vi "ProyectoIII.vi"() -> ()   [LabVIEW 2018]
panel:
  out "Numeric":i64
  out "MEMORY MAP":string[](array[string])
  out "Finished Job Table":string[][](table)
  out "USING DISK":string
  out "NEW":string[](array[string])
  out "RUNNING":string
  out "Program Control Block":string[][](table)
  in  "Address Probability (%)":i32(slide)=64 scale=0.0..100.0
  in  "Page Frames (KB)":i32(slide) step=4 scale=4.0..64.0
  in  "RAM (KB)":i32(slide)=64 step=4 scale=32.0..256.0
  out "WAITING DISK":string[](array[string])
  out "Table Allocation Page":string[][](table)
  in  "Play/Pause":bool
  in  "JOBS":i32=20
  out "I/O WAITING":string[](array[string])
  out "PRINT":string
  out "TERMINATED":string[](array[string])
  out "READY":string[](array[string])
  in  "?":bool
  in  "Delay (s)":sgl(slide) scale=0.0..6.0
  in  "Average Printing Time":i32(slide) scale=10.0..80.0
  in  "Print Probability %":i32(slide) scale=0.0..100.0
  in  "Average Process Time":i32(slide) scale=5.0..100.0
  in  "Quantum":i32(slide) scale=0.0..20.0
  in  "Job Probability %":i32(slide) scale=0.0..100.0
  out "Tiempo imprimiendo":i32
  out "quantum":i32
  out "CLOCK":i32
  # "MEMORY AND PROCESS MANAGER"
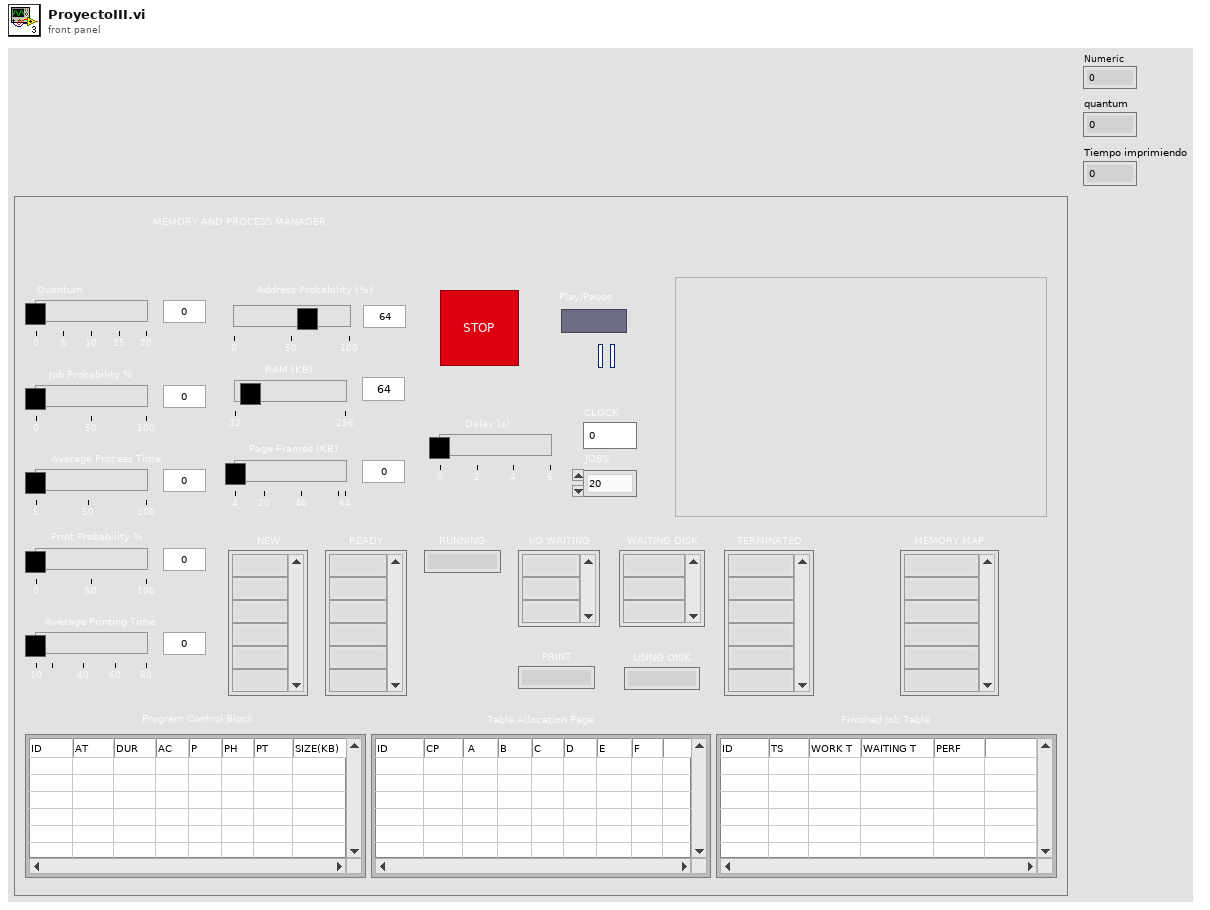
[diagram p1: front panel]
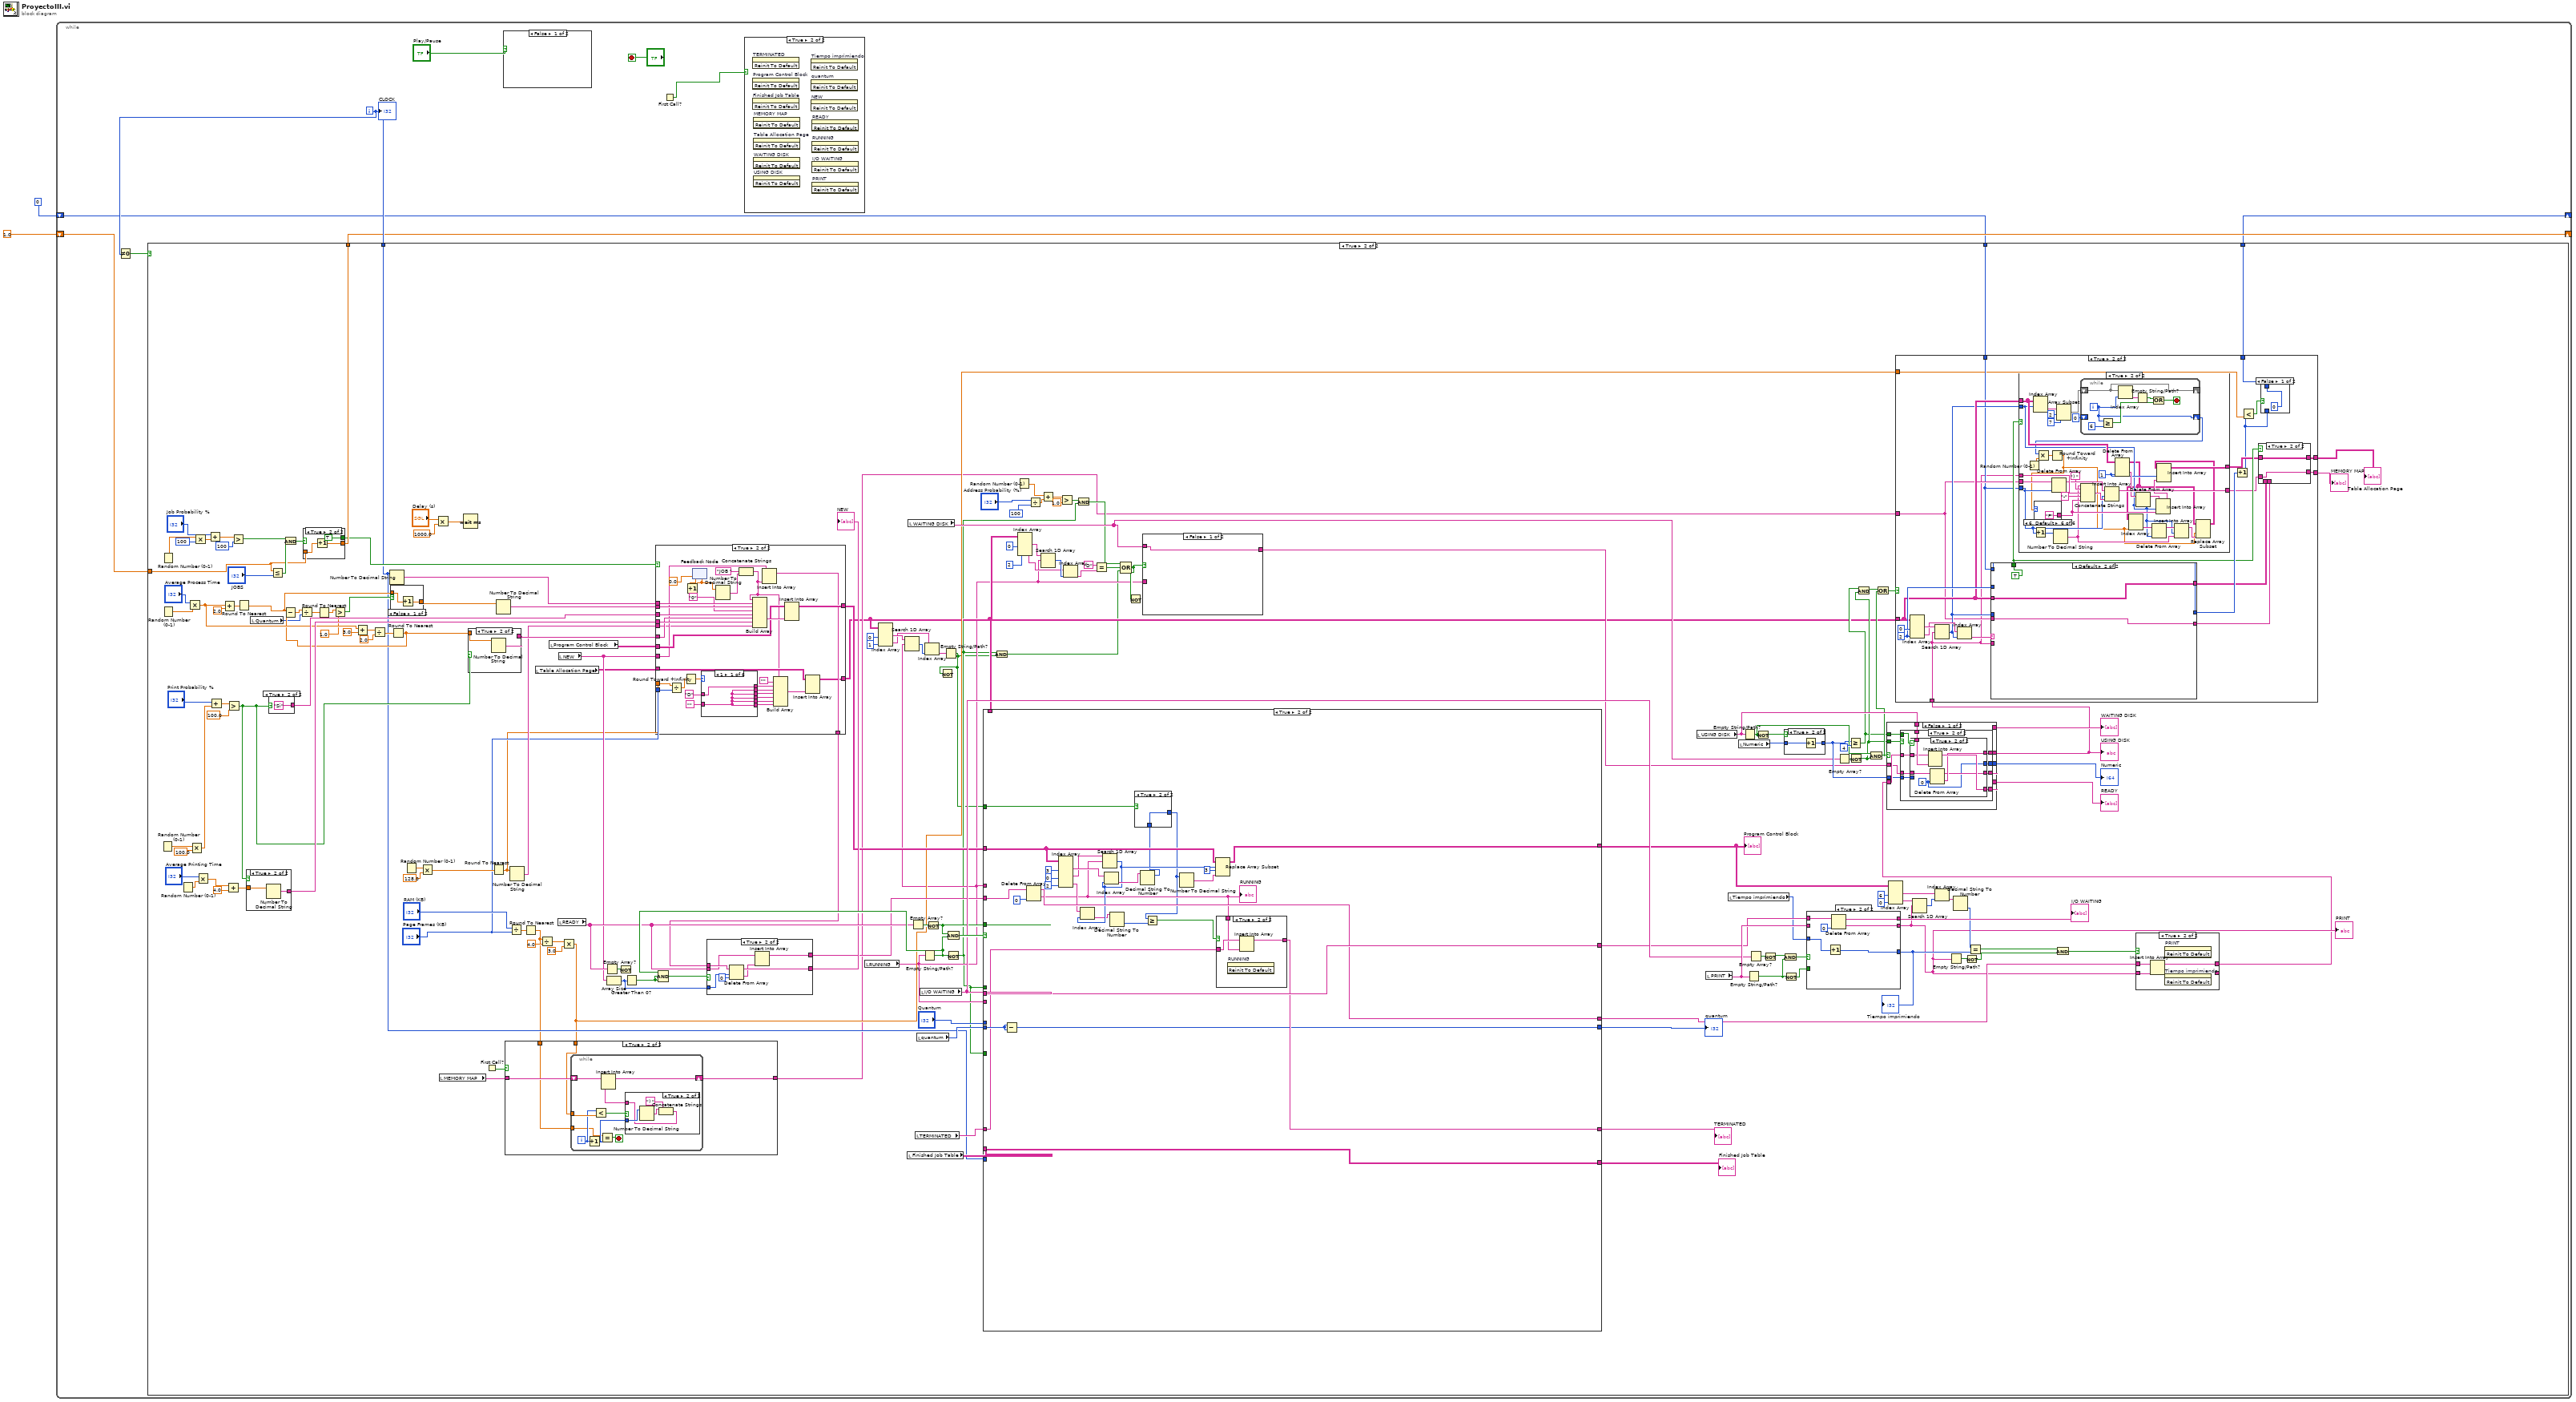
[diagram p0: block diagram]
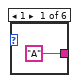
[diagram p8: hidden frame]
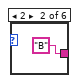
[diagram p9: hidden frame]
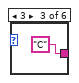
[diagram p10: hidden frame]
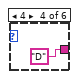
[diagram p11: hidden frame]
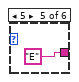
[diagram p12: hidden frame]
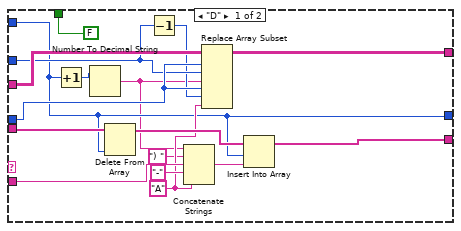
[diagram p13: hidden frame]
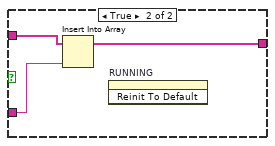
[diagram p14: hidden frame]
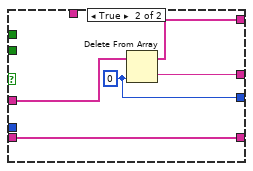
[diagram p17: hidden frame]
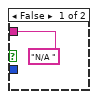
[diagram p20: hidden frame]
diagram:
  n1 = while {
    shift-right: [w6] -> _
    shift-left: 1.0 -> [w7]
    shift-right: [w4] -> _
    shift-left: 0 -> [w5]
    i -> [w8]
    stop <- "?" stop-if-true
    n2 = Not Equal To 0?(x=w8) -> (x != 0?=w9:bool)
    n3 = case shown="True" w9 {
      tunnel: w8 -> [_ w56]
      tunnel: w7 -> [_ w87]
      tunnel: [_ w86] -> w6
      tunnel: w5 -> [w12 w42]
      tunnel: [w12 w40] -> w4
      frame False {
      }
      frame True {
        n4 = Random Number (0-1)() -> (number: 0 to 1=w165:dbl)
        n5 = Random Number (0-1)() -> (number: 0 to 1=w168:dbl)
        n6 = Random Number (0-1)() -> (number: 0 to 1=w171:dbl)
        n7 = Random Number (0-1)() -> (number: 0 to 1=w170:dbl)
        n8 = Multiply(x="Average Process Time", y=w171) -> (x*y=w123:dbl)
        n9 = Multiply(x=w165, y=100.0) -> (x*y=w163:dbl)
        n10 = Multiply(x=w168, y=100) -> (x*y=w166:dbl)
        n11 = Multiply(x="Average Printing Time", y=w170) -> (x*y=w115:dbl)
        n12 = Add(x="Job Probability %", y=w166) -> (x+y=w92:dbl)
        n13 = Add(x="Print Probability %", y=w163) -> (x+y=w178:dbl)
        n14 = Add(x=w123, y=2.0) -> (x+y=w125:dbl)
        n15 = Add(x=w115, y=4.0) -> (x+y=w114:dbl)
        n16 = Greater?(x=w178, y=100.0) -> (0:w157:bool)
        n17 = Greater?(x=w92, y=100) -> (0:w89:bool)
        n18 = Round To Nearest(number=w125) -> (nearest integer value=w95:dbl)
        n19 = case shown="True" w157 {
          tunnel: w114 -> [_ w385]
          tunnel: ["" w384] -> w169
          frame False {
          }
          frame True {
            n20 = Number To Decimal String(number=w385) -> (decimal integer string=w384:string)  [unwired: 1 in]
          }
        }
        n21 = local read "Quantum"() -> (w101:i32)
        n22 = case shown="True" w157 {
          tunnel: ["No" "Si"] -> w172
          frame False {
          }
          frame True {
          }
        }
        n23 = Less Or Equal?(x=w87, y="JOBS") -> (x <= y?=w90:bool)
        n24 = And(x=w89, y=w90) -> (x .and. y?=w88:bool)
        n25 = case shown="True" w88 {
          tunnel: w87 -> [w345 w348]
          tunnel: [w345 w347] -> w86
          tunnel: [FALSE TRUE] -> w78
          frame False {
          }
          frame True {
            n26 = Increment(x=w348) -> (x+1=w347:dbl)
          }
        }
        n27 = Add(x=w123, y=3.0 ("x+y")) -> (x+y=w160:dbl)
        n28 = Divide(x=w160, y=2.0) -> (x/y=w158:dbl)
        n29 = Number To Decimal String(number=w56) -> (decimal integer string=w174:string)  [unwired: 1 in]
        n30 = Round To Nearest(number=w158) -> (nearest integer value=w102:dbl)
        n31 = Subtract(x=w95, y=w102) -> (x-y=w100:dbl)
        n32 = Divide(x=w100, y=w101) -> (x/y=w99:dbl)
        n33 = Round To Nearest(number=w99) -> (nearest integer value=w98:dbl)
        n34 = Greater?(x=w98, y=1.0) -> (0:w96:bool)
        n35 = case shown="False" w96 {
          tunnel: w95 -> [w349 w351]
          tunnel: [w350 w351] -> w94
          frame False {
            n36 = Increment(x=w349) -> (x+1=w350:dbl)
          }
          frame True {
          }
        }
        n37 = Random Number (0-1)() -> (number: 0 to 1=w85:dbl)
        n38 = Multiply(x=w85, y=128.0) -> (x*y=w83:dbl)
        n39 = Multiply(x="Delay (s)", y=1000.0 ("x*y")) -> (x*y=w175:dbl)
        n40 = local read "MEMORY MAP"() -> (w39:string[])
        n41 = Wait (ms)(milliseconds to wait=w175) -> ()  [unwired: 1 out]
        n42 = case shown="True" w157 {
          tunnel: ["" w382] -> w161
          tunnel: w102 -> [_ w381]
          frame False {
          }
          frame True {
            n43 = Number To Decimal String(number=w381) -> (decimal integer string=w382:string)  [unwired: 1 in]
          }
        }
        n44 = First Call?() -> (First Call?: T/F=w38:bool)
        n45 = Round To Nearest(number=w83) -> (nearest integer value=w76:dbl)
        n46 = Number To Decimal String(number=w94) -> (decimal integer string=w173:string)  [unwired: 1 in]
        n47 = Divide(x="RAM (KB)", y="Page Frames (KB)") -> (x/y=w79:dbl)
        n48 = Number To Decimal String(number=w76) -> (decimal integer string=w82:string)  [unwired: 1 in]
        n49 = Round To Nearest(number=w79) -> (nearest integer value=w29:dbl)
        n50 = local read "Table Allocation Page"() -> (w75:string[][])
        n51 = Divide(x=w29, y=4.0) -> (x/y=w32:dbl)
        n52 = local read "Program Control Block"() -> (w155:string[][])
        n53 = local read "READY"() -> (w107:string[])
        n54 = local read "NEW"() -> (w104:string[])
        n55 = Multiply(x=w32, y=3.0) -> (x*y=w27:dbl)
        n56 = case shown="True" w38 {
          tunnel: w39 -> [w325 w329]
          tunnel: [w325 w328] -> w25
          tunnel: w27 -> [_ w327]
          tunnel: w29 -> [_ w326]
          frame False {
          }
          frame True {
            n57 = while {
              tunnel: w327 -> [w336]
              shift-right: [w331] -> w328
              shift-left: w329 -> [w332]
              tunnel: w326 -> [w330]
              i -> [w334]
              stop <- w338 stop-if-true
              n58 = Increment(x=w334) -> (x+1=w333:i32)
              n59 = Less?(x=w334, y=w336) -> (x < y?=w335:bool)
              n60 = Equal?(x=w330, y=w333) -> (x = y?=w338:bool)
              n61 = case shown="True" w335 {
                tunnel: ["N/A " w340] -> w337
                tunnel: w333 -> [_ w343]
                frame False {
                }
                frame True {
                  n62 = Number To Decimal String(number=w343) -> (decimal integer string=w342:string)  [unwired: 1 in]
                  n63 = Concatenate Strings(w342, ") " ("string")) -> (w340:string)
                }
              }
              n64 = Insert Into Array(array=w332, new element=w337) -> (w331:string[])  [unwired: 1 in]
            }
          }
        }
        n65 = Empty Array?(array=w107) -> (empty?=w109:bool)
        n66 = Array Size(array=w104) -> (size(s)=w106:i32)
        n67 = Not(x=w109) -> ()  [unwired: 1 out]
        n68 = Greater Than 0?(x=w106) -> (x > 0?=w103:bool)
        n69 = case shown="True" w78 {
          tunnel: w174 -> [_ w417]
          tunnel: w173 -> [_ w416]
          tunnel: [w387 w421] -> w72
          tunnel: w172 -> [_ w414]
          tunnel: w169 -> [_ w413]
          tunnel: w161 -> [_ w412]
          tunnel: w155 -> [w387 w411]
          tunnel: w104 -> [w388 w409]
          tunnel: [w388 w408] -> w93
          tunnel: w82 -> [_ w406]
          tunnel: "Page Frames (KB)" -> [_ w404]
          tunnel: w76 -> [_ w403]
          tunnel: w75 -> [w386 w393]
          tunnel: [w386 w391] -> w23
          frame False {
          }
          frame True {
            n70 = Divide(x=w403, y=w404) -> (x/y=w405:dbl)
            n71 = Round Toward +Infinity(x=w405) -> (ceil(x): smallest int >= x=w401:dbl)
            n72 = feedback #1(0.0) -> (w418:dbl)
            n73 = Increment(x=w418) -> (x+1=w419:dbl)
            n74 = feedback-in #1(w419) -> ()
            n75 = case shown="1" w401 {
              tunnel: [w424 w426 w428 w430 w432 w433] -> w390
              tunnel: "D" -> [w424 w426 w428 w430 w432 w433]
              tunnel: "" -> [w423 w425 w427 w429 w431 _]
              tunnel: [w423 w425 w427 w429 w432 w433] -> w395
              tunnel: [w423 w426 w428 w430 w432 w433] -> w398
              tunnel: [w423 w425 w428 w430 w432 w433] -> w397
              tunnel: [w423 w425 w427 w430 w432 w433] -> w396
              tunnel: [w423 w425 w427 w429 w431 w433] -> w394
              frame 1 {
              }
              frame 2 {
              }
              frame 3 {
              }
              frame 4 {
              }
              frame 5 {
              }
              frame 6, Default {
              }
            }
            n76 = Number To Decimal String(number=w418) -> (decimal integer string=w410:string)  [unwired: 1 in]
            n77 = Concatenate Strings("JOB ", w410) -> (w392:string)
            n78 = Build Array(w392, w417, w416, "0", w414, w412, w413, w406) -> (w422:string[])
            n79 = Insert Into Array(array=w409, new element=w392) -> (w408:string[])  [unwired: 1 in]
            n80 = Build Array(w392, "", w390, w398, w397, w396, w395, w394) -> (w402:string[])
            n81 = Insert Into Array(array=w411, new element=w422) -> (w421:string[][])  [unwired: 2 in]
            n82 = Insert Into Array(array=w393, new element=w402) -> (w391:string[][])  [unwired: 2 in]
          }
        }
        n83 = local read "RUNNING"() -> (w19:string)
        n84 = Index Array(array=w23, index (col) #1=0 ("disabled index (col)"), index (col) #2=1 ("index (col)")) -> (element #1=w20:string[], element #2=w17:string[])  [unwired: 2 in]
        n85 = Search 1D Array(1D array=w20, element=w19) -> (index of element=w18:i32)  [unwired: 1 in]
        n86 = local read "Finished Job Table"() -> (w112:string[][])
        n87 = local read "WAITING DISK"() -> (w47:string[])
        n88 = Empty Array?(array=w107) -> (empty?=w162:bool)
        n89 = local read "TERMINATED"() -> (w127:string[])
        n90 = local read "quantum"() -> (w145:i32)
        n91 = local read "I/O WAITING"() -> (w150:string[])
        n92 = Empty String/Path?(string/path=w19) -> (empty?=w108:bool)
        n93 = Compound Arithmetic op=AND(w108, w103, w103) -> (w110:bool)
        n94 = case shown="True" w110 {
          tunnel: w107 -> [w352 w356]
          tunnel: w93 -> [w353 w360]
          tunnel: w106 -> [_ w359]
          tunnel: [w353 w358] -> w105
          tunnel: [w352 w355] -> w67
          frame False {
          }
          frame True {
            n95 = Delete From Array(array=w360, length=w359, index=0) -> (deleted portion=w357:string[], array with subset deleted=w358:string[])
            n96 = Insert Into Array(array=w356, new element=w357) -> (w355:string[])  [unwired: 1 in]
          }
        }
        "NEW" <- w105
        n97 = Index Array(array=w17, index=w18) -> (element=w16:string)
        n98 = Not(x=w162) -> (.not. x?=w147:bool)
        n99 = Empty String/Path?(string/path=w16) -> (empty?=w13:bool)
        n100 = Not(x=w13) -> ()  [unwired: 1 out]
        n101 = Not(x=w108) -> (.not. x?=w15:bool)
        n102 = Compound Arithmetic op=AND(w147, w108) -> (w156:bool)
        n103 = case shown="True" w156 {
          tunnel: w67 -> [w479 w602]
          tunnel: w19 -> [w485 _]
          tunnel: w72 -> [w463 w594]
          tunnel: [w462 w593] -> w81
          tunnel: w150 -> [w486 w592]
          tunnel: [w484 w592] -> w149
          tunnel: w15 -> [w480 _]
          tunnel: [w438 w591] -> w128
          tunnel: w19 -> [w436 _]
          tunnel: w145 -> [w443 w590]
          tunnel: "Quantum" -> [w477 _]
          tunnel: [w474 w579] -> w146
          tunnel: w15 -> [w478 _]
          tunnel: w147 -> [w476 _]
          tunnel: w127 -> [w468 w583]
          tunnel: [w467 w582] -> w126
          tunnel: w112 -> [w460 w581]
          tunnel: w56 -> [w459 _]
          tunnel: [w456 w581] -> w111
          tunnel: w23 -> [_ _]
          tunnel: w13 -> [_ w578]
          frame False {
            n104 = Increment(x=w443) -> (x+1=w444:i32)
            n105 = Less Or Equal?(x=w477, y=w444) -> (x <= y?=w461:bool)
            n106 = Index Array(array=w463, index (col) #1=0 ("disabled index (col)"), index (col) #2=3 ("index (col)")) -> (element #1=w501:string[], element #2=w500:string[])  [unwired: 2 in]
            n107 = Search 1D Array(1D array=w501, element=w485) -> (index of element=w497:i32)  [unwired: 1 in]
            n108 = Index Array(array=w500, index=w497) -> (element=w499:string)
            n109 = Decimal String To Number(string=w499) -> (number=w442:i32)  [unwired: 2 in, 1 out]
            n110 = Empty String/Path?(string/path=w436) -> (empty?=w466:bool)
            n111 = Increment(x=w442) -> (x+1=w440:i32)
            n112 = Not(x=w466) -> (.not. x?=w465:bool)
            n113 = Number To Decimal String(number=w440) -> (decimal integer string=w496:string)  [unwired: 1 in]
            n114 = Replace Array Subset(array=w463, new element=w496, index (row)=w497, index (col)=3 ("disabled index (col)")) -> (w462:string[][])
            n115 = Index Array(array=w462, index (col) #1=3 ("disabled index (col)"), index (col) #2=0 ("index (col)"), index (col) #3=2 ("index (col)"), index (col) #4=6 ("index (col)"), index (col) #5=1 ("index (col)")) -> (element #1=w470:string[], element #2=w471:string[], element #3=w454:string[], element #4=w453:string[], element #5=w451:string[])  [unwired: 5 in]
            n116 = Index Array(array=w462, index (col) #1=3 ("disabled index (col)"), index (col) #2=0 ("disabled index (col)"), index (col) #3=5 ("index (col)")) -> (element #1=w493:string[], element #2=w482:string[], element #3=w483:string[])  [unwired: 3 in]
            n117 = Search 1D Array(1D array=w482, element=w485) -> (index of element=w489:i32)  [unwired: 1 in]
            n118 = Search 1D Array(1D array=w471, element=w436) -> (index of element=w445:i32)  [unwired: 1 in]
            n119 = Index Array(array=w454, index=w445) -> (element=w441:string)
            n120 = Index Array(array=w470, index=w445) -> (element=w439:string)
            n121 = Index Array(array=w483, index=w489) -> (element=w488:string)
            n122 = Index Array(array=w493, index=w489) -> (element=w492:string)
            n123 = Decimal String To Number(string=w488) -> (number=w487:i32)  [unwired: 2 in, 1 out]
            n124 = Decimal String To Number(string=w492) -> (number=w491:i32)  [unwired: 2 in, 1 out]
            n125 = Equal?(x=w439, y=w441) -> (x = y?=w464:bool)
            n126 = Equal?(x=w487, y=w491) -> (x = y?=w475:bool)
            n127 = Compound Arithmetic op=AND(w464, w465) -> (w437:bool)
            n128 = Not(x=w437) -> (.not. x?=w448:bool)
            n129 = Compound Arithmetic op=AND(w461, w448) -> (w447:bool)
            n130 = Not(x=w447) -> (.not. x?=w446:bool)
            n131 = case shown="True" w447 {
              tunnel: w436 -> [_ w571]
              tunnel: w479 -> [w560 w570]
              tunnel: [w560 w569] -> w438
              tunnel: w476 -> [w562 _]
              tunnel: w478 -> [w559 _]
              tunnel: w443 -> [w558 w568]
              tunnel: [w557 w567] -> w474
              frame False {
                n132 = And(x=w562, y=w559) -> (x .and. y?=w561:bool)
                n133 = case shown="False" w561 {
                  tunnel: w558 -> [w564 w566]
                  tunnel: [w563 w565] -> w557
                  frame False {
                    n134 = Subtract(x=w564, y=w564) -> (x-y=w563:i32)
                  }
                  frame True {
                    n135 = Increment(x=w566) -> (x+1=w565:i32)
                  }
                }
              }
              frame True {
                n136 = Insert Into Array(array=w570, new element=w571) -> (w569:string[])  [unwired: 1 in]
                n137 = Subtract(x=w568, y=w568) -> (x-y=w567:i32)
              }
            }
            n138 = Compound Arithmetic op=AND(w475, w480, w448, w446) -> (w449:bool)
            n139 = case shown="True" w437 {
              tunnel: w468 -> [w534 w556]
              tunnel: w436 -> [w531 w535]
              tunnel: [w534 w555] -> w467
              tunnel: w460 -> [w533 w539]
              tunnel: w459 -> [_ w554]
              tunnel: w451 -> [_ w553]
              tunnel: w445 -> [_ w552]
              tunnel: w441 -> [w532 w537]
              tunnel: w453 -> [_ w546]
              tunnel: w445 -> [_ w545]
              tunnel: [w533 w540] -> w457
              tunnel: [w532 w537] -> w455
              tunnel: [w531 w535] -> w450
              tunnel: w436 -> [_ _]
              frame False {
              }
              frame True {
                w536 = "" ("element")
                n140 = Index Array(array=w546, index=w545) -> (element=w544:string)
                n141 = Decimal String To Number(string=w537) -> (number=w547:i32)  [unwired: 2 in, 1 out]
                n142 = Index Array(array=w553, index=w552) -> (element=w551:string)
                n143 = Insert Into Array(array=w556, new element=w535) -> (w555:string[])  [unwired: 1 in]
                n144 = Decimal String To Number(string=w544) -> (number=w543:i32)  [unwired: 2 in, 1 out]
                n145 = Decimal String To Number(string=w551) -> (number=w550:i32)  [unwired: 2 in, 1 out]
                n146 = Add(x=w547, y=w543) -> (x+y=w542:i32)
                n147 = Subtract(x=w554, y=w550) -> (x-y=w549:i32)
                n148 = Number To Decimal String(number=w542) -> (decimal integer string=w541:string)  [unwired: 1 in]
                n149 = Number To Decimal String(number=w549) -> (decimal integer string=w548:string)  [unwired: 1 in]
                n150 = Build Array(w535, w548, w541, w536, w536) -> (w538:string[])
                n151 = Insert Into Array(array=w539, new element=w538) -> (w540:string[][])  [unwired: 2 in]
              }
            }
            n152 = case shown="True" w449 {
              tunnel: w486 -> [w572 w575]
              tunnel: w485 -> [_ w574]
              tunnel: [w572 w573] -> w484
              frame False {
              }
              frame True {
                n153 = Insert Into Array(array=w575, new element=w574) -> (w573:string[])  [unwired: 1 in]
              }
            }
            n154 = Compound Arithmetic op=OR(w475, w447, w437) -> (w481:bool)
            n155 = case shown="True" w481 {
              frame False {
              }
              frame True {
                n156 = invoke on="RUNNING" class="Str" method="Reinit To Default"() -> ()  [unwired: 3 in, 3 out]
              }
            }
            n157 = case shown="True" w437 {
              tunnel: w457 -> [w504 w529]
              tunnel: [w504 w518] -> w456
              tunnel: w455 -> [_ w530]
              tunnel: w450 -> [_ w527]
              frame False {
              }
              frame True {
                n158 = Decimal String To Number(string=w530) -> (number=w522:i32)  [unwired: 2 in, 1 out]
                n159 = Index Array(array=w529, index (col) #1=1 ("disabled index (col)"), index (col) #2=0 ("index (col)"), index (col) #3=2 ("index (col)")) -> (element #1=w524:string[], element #2=w525:string[], element #3=w516:string[])  [unwired: 3 in]
                n160 = Search 1D Array(1D array=w525, element=w527) -> (index of element=w511:i32)  [unwired: 1 in]
                n161 = Index Array(array=w516, index=w511) -> (element=w515:string)
                n162 = Index Array(array=w524, index=w511) -> (element=w523:string)
                n163 = Decimal String To Number(string=w515) -> (number=w514:i32)  [unwired: 2 in, 1 out]
                n164 = Decimal String To Number(string=w523) -> (number=w513:i32)  [unwired: 2 in, 1 out]
                n165 = Divide(x=w514, y=w513) -> (x/y=w510:dbl)
                n166 = Subtract(x=w513, y=w522) -> (x-y=w521:i32)
                n167 = Multiply(x=w510, y=100.0) -> (x*y=w508:dbl)
                n168 = Number To Decimal String(number=w521) -> (decimal integer string=w520:string)  [unwired: 1 in]
                n169 = Number To Decimal String(number=w508) -> (decimal integer string=w507:string)  [unwired: 1 in]
                n170 = Concatenate Strings(w507, " %" ("string")) -> (w505:string)
                n171 = Replace Array Subset(array=w529, new element #1=w520, index (row) #1=w511, index (col) #1=3 ("disabled index (col)"), new element #2=w505, index (row) #2=w511, index (col) #2=4 ("index (col)")) -> (w518:string[][])
              }
            }
          }
          frame True {
            n172 = Subtract(x=w590, y=w590) -> (x-y=w579:i32)
            n173 = Delete From Array(array=w602, index=0) -> (deleted portion=w580:string, array with subset deleted=w591:string[])  [unwired: 1 in]
            "RUNNING" <- w580
            n174 = Index Array(array=w594, index (col) #1=3 ("disabled index (col)"), index (col) #2=0 ("index (col)"), index (col) #3=2 ("index (col)")) -> (element #1=w599:string[], element #2=w598:string[], element #3=w588:string[])  [unwired: 3 in]
            n175 = Search 1D Array(1D array=w598, element=w580) -> (index of element=w587:i32)  [unwired: 1 in]
            n176 = Index Array(array=w588, index=w587) -> (element=w586:string)
            n177 = Index Array(array=w599, index=w587) -> (element=w597:string)
            n178 = Decimal String To Number(string=w586) -> (number=w585:i32)  [unwired: 2 in, 1 out]
            n179 = Decimal String To Number(string=w597) -> (offset past number=w577:i32)  [unwired: 2 in, 1 out]
            n180 = case shown="True" w578 {
              tunnel: w577 -> [w604 w606]
              tunnel: [w605 w606] -> w576
              frame False {
                n181 = Increment(x=w604) -> (x+1=w605:i32)
              }
              frame True {
              }
            }
            n182 = Greater Or Equal?(x=w576, y=w585) -> (x >= y?=w584:bool)
            n183 = Number To Decimal String(number=w576) -> (decimal integer string=w595:string)  [unwired: 1 in]
            n184 = Replace Array Subset(array=w594, new element=w595, index (row)=w587, index (col)=3 ("disabled index (col)")) -> (w593:string[][])
            n185 = case shown="True" w584 {
              tunnel: w583 -> [w607 w610]
              tunnel: w580 -> [_ w609]
              tunnel: [w607 w608] -> w582
              frame False {
              }
              frame True {
                n186 = invoke on="RUNNING" class="Str" method="Reinit To Default"() -> ()  [unwired: 3 in, 3 out]
                n187 = Insert Into Array(array=w610, new element=w609) -> (w608:string[])  [unwired: 1 in]
              }
            }
          }
        }
        "Program Control Block" <- w81
        "quantum" <- w146
        "TERMINATED" <- w126
        "Finished Job Table" <- w111
        n188 = And(x=w15, y=w13) -> (x .and. y?=w14:bool)
        n189 = Random Number (0-1)() -> (number: 0 to 1=w74:dbl)
        n190 = Index Array(array=w23, index (col) #1=0 ("index (col)"), index (col) #2=2 ("index (col)")) -> (element #1=w51:string[], element #2=w52:string[])  [unwired: 2 in]
        n191 = Divide(x="Address Probability (%)", y=100) -> (x/y=w69:dbl)
        n192 = Add(x=w74, y=w69) -> (x+y=w73:dbl)
        n193 = Search 1D Array(1D array=w51, element=w19) -> (index of element=w53:i32)  [unwired: 1 in]
        n194 = Greater?(x=w73, y=1.0) -> (0:w46:bool)
        n195 = Index Array(array=w52, index=w53) -> (element=w54:string)
        n196 = And(x=w46, y=w15) -> (x .and. y?=w45:bool)
        n197 = Equal?(x="D", y=w54) -> (x = y?=w44:bool)
        n198 = Compound Arithmetic op=OR(w45, w44, w14) -> (w24:bool)
        n199 = Not(x=w24) -> ()  [unwired: 1 out]
        n200 = case shown="False" w24 {
          tunnel: w19 -> [_ w282]
          tunnel: [w279 w281] -> w48
          tunnel: w47 -> [w279 w280]
          frame False {
          }
          frame True {
            n201 = Insert Into Array(array=w280, new element=w282) -> (w281:string[])  [unwired: 1 in]
            n202 = invoke on="RUNNING" class="Str" method="Reinit To Default"() -> ()  [unwired: 3 in, 3 out]
          }
        }
        n203 = local read "USING DISK"() -> (w60:string)
        n204 = local read "PRINT"() -> (w151:string)
        n205 = local read "Tiempo imprimiendo"() -> (w144:i32)
        n206 = local read "Numeric"() -> (w65:i64)
        n207 = Empty String/Path?(string/path=w60) -> (empty?=w61:bool)
        n208 = Empty String/Path?(string/path=w151) -> (empty?=w134:bool)
        n209 = Empty Array?(array=w150) -> (empty?=w153:bool)
        n210 = Not(x=w61) -> (.not. x?=w34:bool)
        n211 = Not(x=w153) -> (.not. x?=w152:bool)
        n212 = And(x=w152, y=w134) -> (x .and. y?=w135:bool)
        n213 = case shown="True" w34 {
          tunnel: w65 -> [w322 w324]
          tunnel: [w322 w323] -> w57
          frame False {
          }
          frame True {
            n214 = Increment(x=w324) -> (x+1=w323:i64)
          }
        }
        n215 = Not(x=w134) -> (.not. x?=w133:bool)
        n216 = case shown="True" w135 {
          tunnel: w149 -> [w369 w379]
          tunnel: [w370 w378] -> w116
          tunnel: w151 -> [w370 _]
          tunnel: [w369 w377] -> w148
          tunnel: w144 -> [w367 w375]
          tunnel: [w366 w374] -> w136
          tunnel: w133 -> [w368 _]
          frame False {
            n217 = case shown="True" w368 {
              tunnel: w367 -> [w371 w373]
              tunnel: [w371 w372] -> w366
              frame False {
              }
              frame True {
                n218 = Increment(x=w373) -> (x+1=w372:i32)
              }
            }
          }
          frame True {
            n219 = Increment(x=w375) -> (x+1=w374:i32)
            n220 = Delete From Array(array=w379, index=0) -> (deleted portion=w378:string, array with subset deleted=w377:string[])  [unwired: 1 in]
          }
        }
        "I/O WAITING" <- w148
        "PRINT" <- w116
        "Tiempo imprimiendo" <- w136
        n221 = Empty Array?(array=w47) -> (empty?=w66:bool)
        n222 = Greater Or Equal?(x=w57, y=i64 4) -> (x >= y?=w26:bool)
        n223 = Not(x=w66) -> (.not. x?=w33:bool)
        n224 = Compound Arithmetic op=AND(w26, w33) -> (w37:bool)
        n225 = And(x=w61, y=w33) -> (x .and. y?=w36:bool)
        n226 = Or(x=w36, y=w37) -> (x .or. y?=w35:bool)
        n227 = Index Array(array=w81, index (col) #1=6 ("disabled index (col)"), index (col) #2=0 ("index (col)")) -> (element #1=w139:string[], element #2=w141:string[])  [unwired: 2 in]
        n228 = Search 1D Array(1D array=w141, element=w116) -> (index of element=w140:i32)  [unwired: 1 in]
        n229 = Index Array(array=w139, index=w140) -> (element=w138:string)
        n230 = Empty String/Path?(string/path=w116) -> (empty?=w132:bool)
        n231 = Decimal String To Number(string=w138) -> (number=w137:i32)  [unwired: 2 in, 1 out]
        n232 = Not(x=w132) -> (.not. x?=w129:bool)
        n233 = Equal?(x=w137, y=w136) -> (x = y?=w131:bool)
        n234 = And(x=w131, y=w129) -> (x .and. y?=w130:bool)
        n235 = case shown="True" w130 {
          tunnel: w128 -> [w362 w365]
          tunnel: w116 -> [w361 w364]
          tunnel: [w362 w363] -> w59
          tunnel: [w361 _] -> _
          frame False {
          }
          frame True {
            n236 = Insert Into Array(array=w365, new element=w364) -> (w363:string[])  [unwired: 1 in]
            n237 = invoke on="PRINT" class="Str" method="Reinit To Default"() -> ()  [unwired: 3 in, 3 out]
            n238 = invoke on="Tiempo imprimiendo" class="DigNum (strict)" method="Reinit To Default"() -> ()  [unwired: 3 in, 3 out]
          }
        }
        n239 = case shown="False" w36 {
          tunnel: w48 -> [w287 w321]
          tunnel: [w286 w320] -> w43
          tunnel: [w285 w319] -> w63
          tunnel: [w284 w318] -> w62
          tunnel: w33 -> [w292 _]
          tunnel: w26 -> [w291 _]
          tunnel: w60 -> [w290 _]
          tunnel: w59 -> [w289 w317]
          tunnel: [w288 w317] -> w58
          tunnel: w57 -> [w283 _]
          frame False {
            n240 = case shown="True" w292 {
              tunnel: w291 -> [_ w305]
              tunnel: w290 -> [w294 w304]
              tunnel: w289 -> [w295 w303]
              tunnel: [w295 w302] -> w288
              tunnel: w287 -> [w296 w301]
              tunnel: [w294 w300] -> w286
              tunnel: [w296 w299] -> w285
              tunnel: [w293 w298] -> w284
              tunnel: w283 -> [w293 w297]
              frame False {
              }
              frame True {
                n241 = case shown="True" w305 {
                  tunnel: w304 -> [w309 w316]
                  tunnel: w303 -> [w308 w315]
                  tunnel: [w308 w314] -> w302
                  tunnel: w301 -> [w307 w313]
                  tunnel: [w309 w312] -> w300
                  tunnel: [w307 w311] -> w299
                  tunnel: [w306 w310] -> w298
                  tunnel: w297 -> [w306 _]
                  frame False {
                  }
                  frame True {
                    w310 = 0 ("index")
                    n242 = Insert Into Array(array=w315, new element=w316) -> (w314:string[])  [unwired: 1 in]
                    n243 = Delete From Array(array=w313, index=w310) -> (deleted portion=w312:string, array with subset deleted=w311:string[])  [unwired: 1 in]
                  }
                }
              }
            }
          }
          frame True {
            w318 = 0 ("index")
            n244 = Delete From Array(array=w321, index=w318) -> (deleted portion=w320:string, array with subset deleted=w319:string[])  [unwired: 1 in]
          }
        }
        "READY" <- w58
        "USING DISK" <- w43
        "WAITING DISK" <- w63
        "Numeric" <- w62
        n245 = case shown="True" w35 {
          tunnel: w23 -> [w180 w198]
          tunnel: w43 -> [_ w189]
          tunnel: w42 -> [w181 w190]
          tunnel: w25 -> [w182 w191]
          tunnel: [w182 w187] -> w41
          tunnel: [w181 w184] -> w40
          tunnel: [w180 w194] -> w28
          tunnel: w27 -> [_ w183]
          frame False {
          }
          frame True {
            w200 = 2 ("index (col)")
            n246 = Index Array(array=w198, index (col) #1=0 ("disabled index (col)"), index (col) #2=w200) -> (element #1=w202:string[], element #2=w201:string[])  [unwired: 2 in]
            n247 = Search 1D Array(1D array=w202, element=w189) -> (index of element=w197:i32)  [unwired: 1 in]
            n248 = Index Array(array=w201, index=w197) -> (element=w203:string)
            n249 = case shown="Default" w203 {
              tunnel: w198 -> [w268 w278]
              tunnel: [w267 w278] -> w193
              tunnel: w190 -> [w260 w276]
              tunnel: w191 -> [w272 w277]
              tunnel: w189 -> [w274 _]
              tunnel: [w270 w277] -> w192
              tunnel: [w260 w276] -> w199
              tunnel: w197 -> [w266 _]
              tunnel: w200 -> [w265 _]
              tunnel: [FALSE TRUE] -> w196
              frame "D" {
                w261 = "A" ("string")
                n250 = Increment(x=w260) -> (x+1=w262:i32)
                n251 = Number To Decimal String(number=w262) -> (decimal integer string=w259:string)  [unwired: 1 in]
                n252 = Delete From Array(array=w272, index=w260) -> (array with subset deleted=w269:string[])  [unwired: 1 in, 1 out]
                n253 = Decrement(x=w265) -> (x-1=w264:i32)
                n254 = Concatenate Strings(w259, ") " ("string"), w274, "-" ("string"), w261) -> (w271:string)
                n255 = Replace Array Subset(array=w268, new element #1=w259, index (row) #1=w266, index (col) #1=w265, new element #2=w261, index (row) #2=w266, index (col) #2=w264) -> (w267:string[][])
                n256 = Insert Into Array(array=w269, index=w260, new element=w271) -> (w270:string[])
              }
              frame Default {
              }
            }
            n257 = case shown="True" w196 {
              tunnel: w198 -> [w212 w239]
              tunnel: w197 -> [_ w220]
              tunnel: [w212 w233] -> w195
              tunnel: w191 -> [w211 w236]
              tunnel: w190 -> [_ w216]
              tunnel: w189 -> [_ w237]
              tunnel: [w211 w234] -> w188
              frame False {
              }
              frame True {
                w231 = 1 ("disabled index (col)")
                n258 = Random Number (0-1)() -> (number: 0 to 1=w241:dbl)
                n259 = Index Array(array=w239, index (row)=w220) -> (element=w244:string[])  [unwired: 1 in]
                n260 = Increment(x=w216) -> (x+1=w229:i32)
                n261 = Delete From Array(array=w236, index=w216) -> (array with subset deleted=w230:string[])  [unwired: 1 in, 1 out]
                n262 = Number To Decimal String(number=w229) -> (decimal integer string=w215:string)  [unwired: 1 in]
                n263 = Array Subset(array=w244, index=2, length=7) -> (w223:string[])
                n264 = while {
                  shift-right: [w256] -> _
                  shift-left: w223 -> [w256]
                  shift-right: [w251] -> w213
                  shift-left: 0 ("y") -> [_]
                  i -> [w251]
                  stop <- w252 stop-if-true
                  n265 = Greater Or Equal?(x=w251, y=6) -> (x >= y?=w253:bool)
                  n266 = Index Array(array=w256, index=w251) -> (element=w255:string)
                  n267 = Empty String/Path?(string/path=w255) -> (empty?=w254:bool)
                  n268 = Or(x=w254, y=w253) -> (x .or. y?=w252:bool)
                }
                n269 = Multiply(x=w213, y=w241) -> (x*y=w240:dbl)
                n270 = Round Toward +Infinity(x=w240) -> (ceil(x): smallest int >= x=w214:dbl)
                n271 = case shown="6, Default" w214 {
                  tunnel: ["A" "B" "C" "D" "E" "F"] -> w225
                  frame 1 {
                  }
                  frame 2 {
                  }
                  frame 3 {
                  }
                  frame 4 {
                  }
                  frame 5 {
                  }
                  frame 6, Default {
                  }
                }
                n272 = Concatenate Strings(w215, ") " ("string"), w237, "-" ("string"), w225) -> (w235:string)
                n273 = Insert Into Array(array=w230, index=w216, new element=w235) -> (w234:string[])
                n274 = Delete From Array(array=w239, index (col)=w231) -> (deleted portion=w232:string[], array with subset deleted=w217:string[][])  [unwired: 2 in]
                n275 = Index Array(array=w217, index (col)=w214) -> (element=w222:string[])  [unwired: 1 in]
                n276 = Delete From Array(array=w232, index=w220) -> (array with subset deleted=w226:string[])  [unwired: 1 in, 1 out]
                n277 = Delete From Array(array=w222, index=w220) -> (array with subset deleted=w221:string[])  [unwired: 1 in, 1 out]
                n278 = Insert Into Array(array=w226, index=w220, new element=w225) -> (w224:string[])
                n279 = Insert Into Array(array=w221, index=w220, new element=w215) -> (w219:string[])
                n280 = Replace Array Subset(array=w217, new element=w219, index (col)=w214) -> (w218:string[][])  [unwired: 1 in]
                n281 = Insert Into Array(array=w218, index (col)=w231, new element=w224) -> (w233:string[][])  [unwired: 1 in]
              }
            }
            n282 = Increment(x=w199) -> (x+1=w185:i32)
            n283 = Less?(x=w185, y=w183) -> (x < y?=w186:bool)
            n284 = case shown="True" w196 {
              tunnel: w195 -> [_ w210]
              tunnel: [w208 w210] -> w194
              tunnel: w193 -> [w208 _]
              tunnel: w192 -> [w207 _]
              tunnel: w188 -> [_ w209]
              tunnel: [w207 w209] -> w187
              frame False {
              }
              frame True {
              }
            }
            n285 = case shown="False" w186 {
              tunnel: w185 -> [_ w206]
              tunnel: [0 ("y") w206] -> w184
              frame False {
              }
              frame True {
              }
            }
          }
        }
        "MEMORY MAP" <- w41
        "Table Allocation Page" <- w28
      }
    }
    n286 = case shown="False" "Play/Pause" {
      frame False {
      }
      frame True {
        n287 = while {
          stop <- w611 continue-if-true
          n288 = local read "Play/Pause"() -> (w611:bool)
          n289 = Wait (ms)(milliseconds to wait=u32 1000) -> ()  [unwired: 1 out]
        }
      }
    }
    n290 = First Call?() -> (First Call?: T/F=w3:bool)
    n291 = case shown="True" w3 {
      frame False {
      }
      frame True {
        n292 = invoke on="TERMINATED" class="Arr (strict)" method="Reinit To Default"() -> ()  [unwired: 3 in, 3 out]
        n293 = invoke on="Program Control Block" class="Tbl (strict)" method="Reinit To Default"() -> ()  [unwired: 3 in, 3 out]
        n294 = invoke on="Finished Job Table" class="Tbl (strict)" method="Reinit To Default"() -> ()  [unwired: 3 in, 3 out]
        n295 = invoke on="MEMORY MAP" class="Arr (strict)" method="Reinit To Default"() -> ()  [unwired: 3 in, 3 out]
        n296 = invoke on="Table Allocation Page" class="Tbl (strict)" method="Reinit To Default"() -> ()  [unwired: 3 in, 3 out]
        n297 = invoke on="WAITING DISK" class="Arr (strict)" method="Reinit To Default"() -> ()  [unwired: 3 in, 3 out]
        n298 = invoke on="USING DISK" class="Str" method="Reinit To Default"() -> ()  [unwired: 3 in, 3 out]
        n299 = invoke on="Tiempo imprimiendo" class="DigNum (strict)" method="Reinit To Default"() -> ()  [unwired: 3 in, 3 out]
        n300 = invoke on="quantum" class="DigNum (strict)" method="Reinit To Default"() -> ()  [unwired: 3 in, 3 out]
        n301 = invoke on="NEW" class="Arr (strict)" method="Reinit To Default"() -> ()  [unwired: 3 in, 3 out]
        n302 = invoke on="READY" class="Arr (strict)" method="Reinit To Default"() -> ()  [unwired: 3 in, 3 out]
        n303 = invoke on="RUNNING" class="Str" method="Reinit To Default"() -> ()  [unwired: 3 in, 3 out]
        n304 = invoke on="I/O WAITING" class="Arr (strict)" method="Reinit To Default"() -> ()  [unwired: 3 in, 3 out]
        n305 = invoke on="PRINT" class="Str" method="Reinit To Default"() -> ()  [unwired: 3 in, 3 out]
      }
    }
    "CLOCK" <- w8
  }
